vi "LVProjectShortcut_Version.vi"() -> (2 "Library Info":T1={"Name"="LabVIEW Shortcut Provider", "Version String"="1.1.0.13", "Copyright"="Copyright (c) 2022, BenjaminR \nAll rights reserved.", "License"="Zero-Clause BSD\nPermission to use, copy, modify, and/or distribute this software for any purpose with or without fee is hereby granted.\n\nTHE SOFTWARE IS PROVIDED \"AS IS\" AND THE AUTHOR DISCLAIMS ALL WARRANTIES WITH REGARD TO THIS SOFTWARE INCLUDING ALL IMPLIED\nWARRANTIES OF MERCHANTABILITY AND FITNESS. IN NO EVENT SHALL THE AUTHOR BE LIABLE FOR ANY SPECIAL, DIRECT, INDIRECT, OR\nCONSEQUENTIAL DAMAGES OR ANY DAMAGES WHATSOEVER RESULTING FROM LOSS OF USE, DATA OR PROFITS, WHETHER IN AN ACTION OF CONTRACT,\nNEGLIGENCE OR OTHER TORTIOUS ACTION, ARISING OUT OF OR IN CONNECTION WITH THE USE OR PERFORMANCE OF THIS SOFTWARE."})   [LabVIEW 2017, in "LVProject Shortcut.lvlib"]
doc: "Returns library version info."
uses:
  LVProject Shortcut.lvlib
panel:
  # "This data is updated during \nthe package pre-build step"
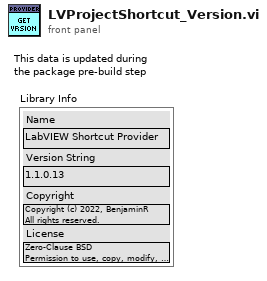
[diagram p1: front panel]
types:
  T1 = cluster{"Name":string, "Version String":string, "Copyright":string, "License":string}
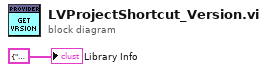
[diagram p0: block diagram]
diagram:
  "Library Info" <- T1 {"Name"="LVProject Shortcut", "Version String"="1.0.1.14", "Copyright"="Copyright (c) 2022, BenjaminR \nAll rights reserved.", "License"="Zero-Clause BSD\nPermission to use, copy, modify, and/or distribute this software for any purpose with or without fee is hereby granted.\n\nTHE SOFTWARE IS PROVIDED \"AS IS\" AND THE AUTHOR DISCLAIMS ALL WARRANTIES WITH REGARD TO THIS SOFTWARE INCLUDING ALL IMPLIED\nWARRANTIES OF MERCHANTABILITY AND FITNESS. IN NO EVENT SHALL THE AUTHOR BE LIABLE FOR ANY SPECIAL, DIRECT, INDIRECT, OR\nCONSEQUENTIAL DAMAGES OR ANY DAMAGES WHATSOEVER RESULTING FROM LOSS OF USE, DATA OR PROFITS, WHETHER IN AN ACTION OF CONTRACT,\nNEGLIGENCE OR OTHER TORTIOUS ACTION, ARISING OUT OF OR IN CONNECTION WITH THE USE OR PERFORMANCE OF THIS SOFTWARE."} ("Library Info Cste")
